vi "Source Compliance Query.vi"(8 "error in (no error)":errorcluster, 9 "Channel (Channel A)":T1, 10 "Node In":string, 11 "VISA resource name":refnum<visa-resource-name>) -> (0 "error out":errorcluster, 1 "Compliance":bool, 2 "Node Out":string, 3 "VISA resource name out":refnum<visa-resource-name>, 4 "Command String":string)   [LabVIEW 2009, in "Keithley 2600 Series.lvlib"]
doc: "This VI querys the SMU source to see if it is in compliance.\n\nIf the source output is being limited by the limit function (in compliance) then Compliance will return true. If the source output is not being limited by the limit function then Compliance will return false.\n\n<b>Functions and Attributes Used</b>\nsmuX.source.compliance"
uses:
  <instrlib>/Keithley 2600 Series/Keithley 2600 Series.lvlib
  <instrlib>/Keithley 2600 Series/Public/Channel.ctl
  <instrlib>/Keithley 2600 Series/Private/GlobalVariables.vi
panel:
  # "(c) 2008 Keithley Instruments, Inc.  ALL RIGHTS RESERVED."
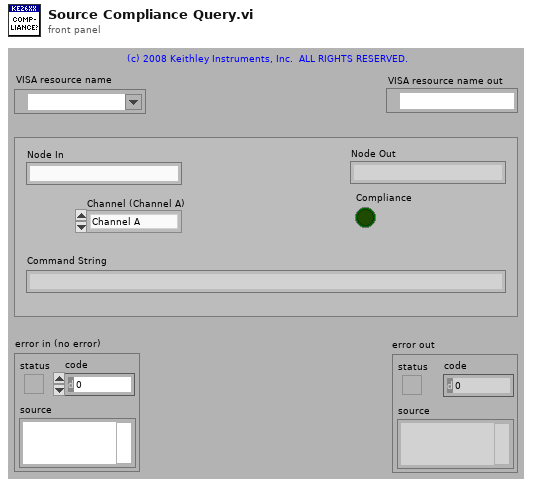
[diagram p1: front panel]
types:
  T1 = typedef "Keithley 2600 Series.lvlib/Channel.ctl" = enum32{"Channel A", "Channel B"}
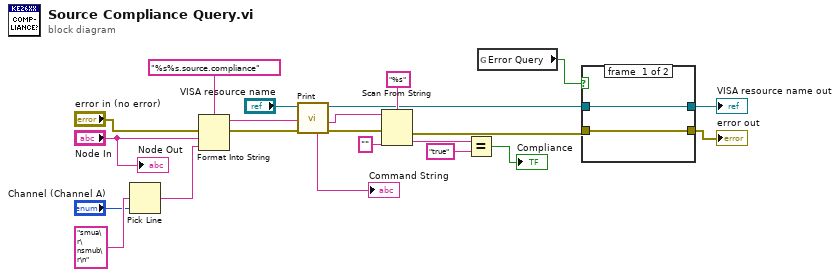
[diagram p0: block diagram]
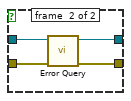
[diagram p2: hidden frame]
diagram:
  n1 = Pick Line(multi-line string="smua\r\nsmub\r\n" ("options"), line index="Channel (Channel A)") -> (output string=w5:string)  [unwired: 1 out]
  n2 = Format Into String(format string="%s%s.source.compliance" ("command"), error in="error in (no error)", "Node In", w5) -> (resulting string=w6:string, error out=w7:errorcluster)  [unwired: 1 in]
  n3 = call <instrlib>:"Print.vi"("error in (no error)"=w7, "Input"=w6, "VISA resource name"="VISA resource name") -> ("error out"=w10:errorcluster, "Output"=w9:string, "VISA resource name out"=w11:refnum<visa-resource-name>, "Command String"=→"Command String":string)  [unwired: 2 in, 3 out]
  n4 = Scan From String(format string="%s", input string=w9, error in=w10, default 1="" ("default value 1")) -> (error out=w14:errorcluster, output 1=w18:string)  [unwired: 1 in, 2 out]
  n5 = Equal?(x=w18, y="true") -> (x = y?=→"Compliance":bool)
  n6 = global read "GlobalVariables.vi" "Error Query"() -> (w15:bool)
  n7 = case shown="True" w15 {
    tunnel: w11 -> [w24 w28]
    tunnel: w14 -> [w23 w27]
    tunnel: [w24 w26] -> w13
    tunnel: [w23 w25] -> w12
    frame #0 {
    }
    frame #1 {
      n8 = call <instrlib>:"Error Query.vi"("error in (no error)"=w27, "VISA resource name"=w28) -> ("error out"=w25:errorcluster, "VISA resource name out"=w26:refnum<visa-resource-name>)  [unwired: 8 out]
    }
  }
  "VISA resource name out" <- w13
  "error out" <- w12
  "Node Out" <- "Node In"
